vi "frequency.vi"(8 "error in (no error)":errorcluster, 10 "Denominator":dbl[](array[numeric]), 11 "Numerator":dbl[](array[numeric])) -> (0 "error out":errorcluster, 1 "s-domain":picture, 2 "Discrete Transfer Function Model":T2 {"transfer function(s)"."delay" format="%.4f"; "transfer function(s)"."Denominator" format="%#_3g"; "transfer function(s)"."Numerator" format="%#_3g"; "properties"."Sampling Time" format="%#.6p"; "properties"."Output Delays" format="%.4f"; "properties"."Input Delays" format="%.4f"}, 3 "transfer function(s)":T1[][](array[typedef]) {"delay" format="%.4f"; "Denominator" format="%#_3g"; "Numerator" format="%#_3g"}, 4 "z-domain":picture, 5 "Step Response Graph":cluster{"time":dbl[], dbl[]}[](array[cluster]), 7 "Transfer Function Model":T2 {"transfer function(s)"."delay" format="%.4f"; "transfer function(s)"."Denominator" format="%#_3g"; "transfer function(s)"."Numerator" format="%#_3g"; "properties"."Sampling Time" format="%#.6p"; "properties"."Output Delays" format="%.4f"; "properties"."Input Delays" format="%.4f"})   [LabVIEW 2022 SP3]
uses:
  <vilib>/addons/Control Design/_Model Construction/Model Typedefs.llb/CD Transfer Function Model (MIMO).ctl
  <vilib>/addons/Control Design/_Model Construction/Model Typedefs.llb/CD General Elements.ctl
  <vilib>/addons/Control Design/_Model Construction/Model Typedefs.llb/CD Transfer Function Model (SISO).ctl
  <vilib>/addons/Control Design/_Model Construction/Data Typedefs.llb/CD CtoD Conversion Method.ctl
  <vilib>/addons/Control Design/_Utility/Rendering.llb/Rendering Transfer Function Options.ctl
  <vilib>/addons/Control Design/_Model Construction/Model Creation.llb/Model Creation SubVI/cd_Create Transfer Function Model.vi
  <vilib>/addons/Control Design/_Time Response Analysis/Time Response.llb/Time Response subVI/cd_Step Response (Transfer Function).vi
  <vilib>/addons/Control Design/_Model Conversions/Continuous and Discrete.llb/Continuous and Discrete SubVI/cd_Convert Continuous to Discrete (TF).vi
  <vilib>/addons/Control Design/_Utility/Model Viewer.llb/Model Viewer SubVI/cd_Draw Transfer Function Equation (TF).vi
  <vilib>/addons/Control Design/_Model Construction/NI_LinSys_Model Creation.lvlib
  <vilib>/addons/Control Design/_Model Conversions/NI_CD_Continuous and Discrete.lvlib
  <vilib>/addons/Control Design/_Model Construction/NI_LinSys_Data Typedefs.lvlib
  <vilib>/addons/Control Design/_Utility/NI_CD_Model Viewer.lvlib
  <vilib>/addons/Control Design/_Utility/NI_LinSys_Rendering.lvlib
  <vilib>/addons/Control Design/_Time Response Analysis/NI_CD_Time Response.lvlib
  <vilib>/addons/Control Design/_Model Construction/NI_LinSys_Model Typedefs.lvlib
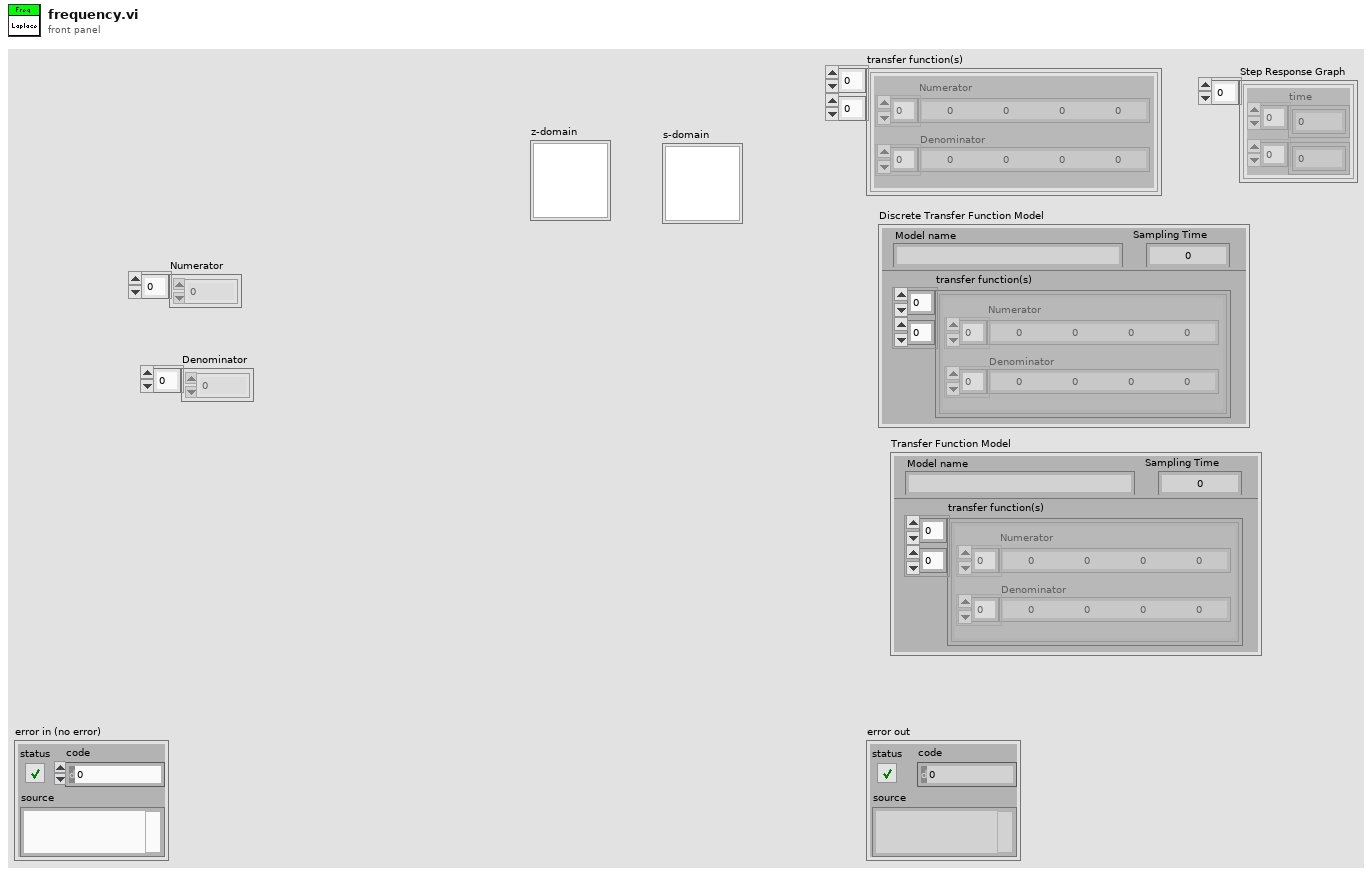
[diagram p1: front panel]
types:
  T1 = typedef "NI_LinSys_Model Typedefs.lvlib/CD Transfer Function Model (SISO).ctl" = cluster{"Numerator":dbl[], "Denominator":dbl[], "delay":dbl}
  T2 = typedef "NI_LinSys_Model Typedefs.lvlib/CD Transfer Function Model (MIMO).ctl" = cluster{"properties":T3, "transfer function(s)":T1[][]}
  T3 = typedef "NI_LinSys_Model Typedefs.lvlib/CD General Elements.ctl" = cluster{"Model name":string, "Input names":string[], "Output names":string[], "Input Delays":dbl[], "Output Delays":dbl[], "Sampling Time":dbl, "Notes":string}
  T4 = typedef "NI_LinSys_Rendering.lvlib/Rendering Transfer Function Options.ctl" = u16
  T5 = typedef "NI_LinSys_Data Typedefs.lvlib/CD CtoD Conversion Method.ctl" = u16
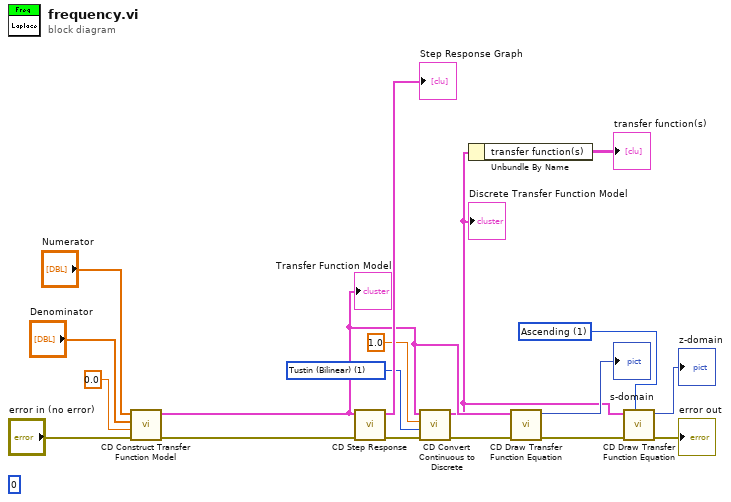
[diagram p0: block diagram]
diagram:
  (unwired) 0 ("index")
  w5 = T4 1 items=["Descending", "Ascending", "Negative Power"] ("Display Format")
  w4 = T5 1 items=["Zero-Order-Hold", "Tustin (Bilinear)", "Prewarp", "Forward", "Backward", "Z-Transform", "First-Order-Hold", "Matched Pole-Zero"] ("Method")
  n1 = call-poly <vilib>:"CD Construct Transfer Function Model.vi"("error in (no error)"="error in (no error)", "Delay"=0.0 ("delay"), "Denominator"="Denominator", "Numerator"="Numerator") -> ("error out"=w13:errorcluster, "Transfer Function Model"=w12:T2)  [unwired: 6 in]
  "Transfer Function Model" <- w12
  n2 = call-poly <vilib>:"CD Step Response.vi"("error in (no error)"=w13, "Transfer Function Model"=w12) -> ("error out"=w14:errorcluster, "Step Response Graph"=→"Step Response Graph":cluster{"time":dbl[], dbl[]}[])  [unwired: 7 in, 1 out]
  n3 = call-poly <vilib>:"CD Convert Continuous to Discrete.vi"("error in (no error)"=w14, "Method"=w4, "Sampling Time (s)"=1.0, "Continuous Transfer Function Model"=w12) -> ("error out"=w10:errorcluster, "Discrete Transfer Function Model"=w8:T2)  [unwired: 6 in]
  "Discrete Transfer Function Model" <- w8
  n4 = Unbundle By Name(w8) -> ("transfer function(s)"=→"transfer function(s)":T1[][])
  n5 = call-poly <vilib>:"CD Draw Transfer Function Equation.vi"("error in (no error)"=w10, "Transfer Function Model"=w12) -> ("error out"=w11:errorcluster, "Equation"=→"s-domain":picture)  [unwired: 7 in, 1 out]
  n6 = call-poly <vilib>:"CD Draw Transfer Function Equation.vi"("Display Format"=w5, "error in (no error)"=w11, "Transfer Function Model"=w8) -> ("error out"=→"error out":errorcluster, "Equation"=→"z-domain":picture)  [unwired: 6 in, 1 out]
